vi "Flatten 2D zero terminated array.vi"(10 "2D zero terminated array":T2(array[cluster])) -> (2 "Flattened Array":T1(array[cluster]))   [LabVIEW 2014, in "Melody Extraction.lvlib"]
uses:
  Melody Extraction.lvlib
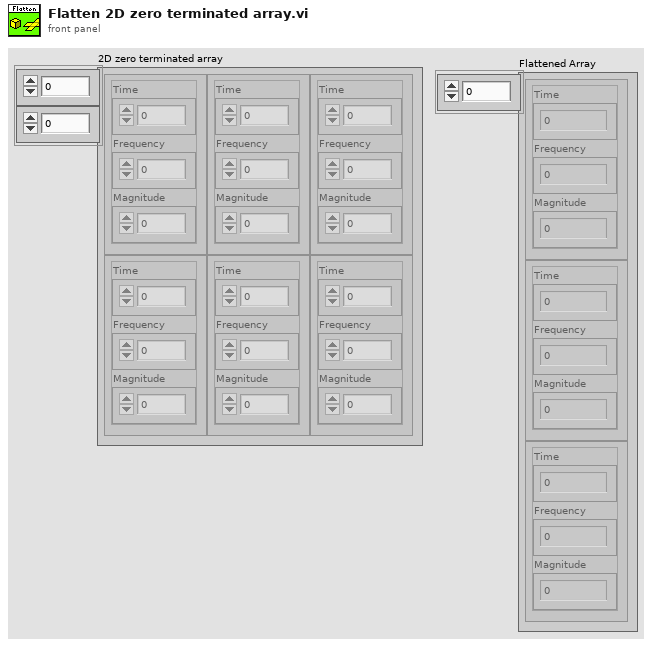
[diagram p1: front panel]
types:
  T1 = cluster{"Time":dbl, "Frequency":dbl, "Magnitude":dbl}[]
  T2 = cluster{"Time":dbl, "Frequency":dbl, "Magnitude":dbl}[][]
  T3 = cluster{"Time":dbl, "Frequency":dbl, "Magnitude":dbl}
  T4 = cluster{"Time":bool, "Frequency":bool, "Magnitude":bool}
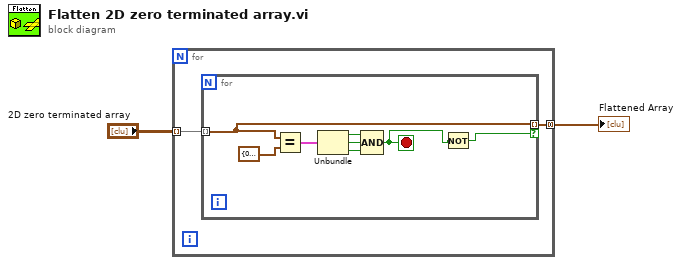
[diagram p0: block diagram]
diagram:
  n1 = for {
    tunnel: "2D zero terminated array" -> [w4] mode=indexing
    tunnel: [w3] -> w1 mode=concatenating
    n2 = for {
      tunnel: w4 -> [w7] mode=indexing
      tunnel: [w7] -> w3 mode=indexing if=w6
      stop <- w5 stop-if-true
      n3 = Equal?(x=w7, y=T3 {"Time"=0.0, "Frequency"=0.0, "Magnitude"=0.0} ("Cluster")) -> (x = y?=w11:T4)
      n4 = Unbundle(w11) -> ("Time"=w10:bool, "Frequency"=w9:bool, "Magnitude"=w8:bool)
      n5 = Compound Arithmetic op=AND(w10, w9, w8) -> (w5:bool)
      n6 = Not(x=w5) -> (.not. x?=w6:bool)
    }
  }
  "Flattened Array" <- w1
